vi "Main.vi"(5 "Amplitude(V)":dbl=5.0 min=-1000000000.0 max=1000000000.0 format="%#_13g", 11 "Error_In":errorcluster) -> (0 "Analog_Waveform":waveform(dbl)(graph)={"t0"=timestamp(0 s since 1904-01-01), "dt"=1e-06, "Y"=array[5000 elements]}, 3 "Min_Peak_Point":dbl format="%0.2f", 4 "Digital_Waveform":digitaldata(graph), 6 "Rise_Time (s)":dbl, 8 "Fall_Time (s)":dbl, 14 "Max_Peak_Point":dbl format="%0.2f", 15 "Error_Out":errorcluster)   [LabVIEW 2021]
doc: "This VI is the main VI which communicate with other SubVIs and Displays the output."
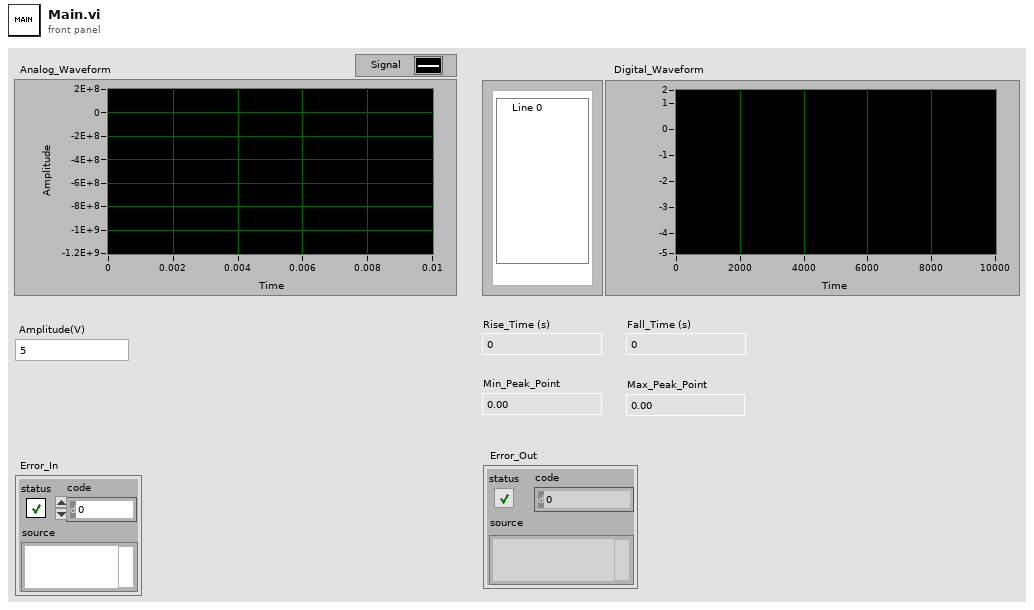
[diagram p1: front panel]
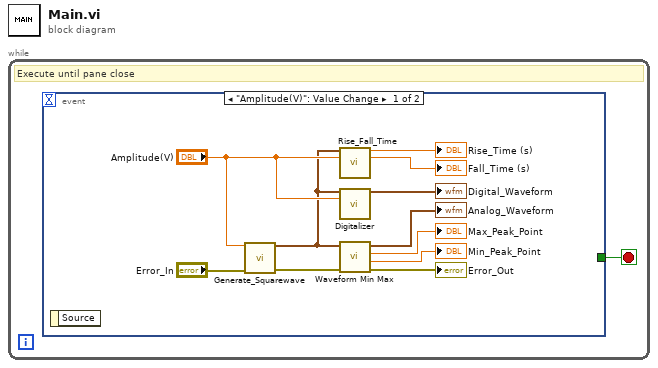
[diagram p0: block diagram]
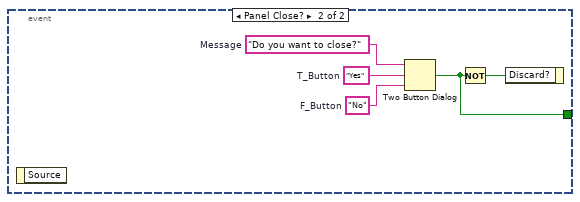
[diagram p2: hidden frame]
diagram:
  n1 = while {
    stop <- w1 stop-if-true
    # "Execute until pane close"
    n2 = event shown="[0] \"Amplitude(V)\": Value Change" {
      selector: _ -> [_ _]
      dyn-events: _ -> [_ _]
      timeout: _ -> [_ _]
      tunnel: [_ w13] -> w1
      event "Amplitude(V)": Value Change {
        n3 = event-data() -> ()  [unwired: 1 in, 1 out]
        n4 = call "Generate_Squarewave.vi"("Amplitude(V)"="Amplitude(V)", "Error_In"="Error_In") -> ("Waveform_Out"=w7:waveform(dbl), "Error_Out"=w6:errorcluster)  [unwired: 12 in]
        n5 = call "Rise_Fall_Time.vi"("Analog_Waveform"=w7, "Amplitude(V)"="Amplitude(V)") -> ("Rise_Time (s)"=→"Rise_Time (s)":dbl, "Fall_Time (s)"=→"Fall_Time (s)":dbl)  [unwired: 12 in]
        n6 = call "Digitalizer.vi"("Analog_Waveform"=w7, "Amplitude(V)"="Amplitude(V)") -> ("Digital_Waveform"=→"Digital_Waveform":digitaldata)  [unwired: 13 in]
        n7 = call <vilib>:"Waveform Min Max.vi"("error in (no error)"=w6, "waveform in"=w7) -> ("error out"=→"Error_Out":errorcluster, "Y min"=→"Min_Peak_Point":dbl, "Y max"=→"Max_Peak_Point":dbl, "waveform out"=→"Analog_Waveform":waveform(dbl))  [unwired: 4 in, 2 out]
      }
      event Panel Close? {
        w15 = "No"  # F_Button
        w16 = "Yes"  # T_Button
        w17 = "Do you want to close?"  # Message
        n8 = event-data() -> ()  [unwired: 1 in, 1 out]
        n9 = Two Button Dialog(message=w17, 1:w15, 2:w16) -> (T button?=w13:bool)
        n10 = Not(x=w13) -> (.not. x?=w14:bool)
        n11 = event-data("Discard?"=w14) -> ()  [unwired: 1 in, 1 out]
      }
    }
  }
